vi "Temperature and Humidity Data Acqusition and Logging.vi"() -> ()   [LabVIEW 2017]
uses:
  <vilib>/Instr/_visa.llb/VISA Configure Serial Port (Instr).vi
  <vilib>/Utility/file.llb/Write Delimited Spreadsheet (string).vi
  <vilib>/regexp/Match Regular Expression.xnode
panel:
  out "read buffer":string
  out "Temperature (°F) 2":i32(slide) scale=0.0..300.0
  out "Temperature (°C) 2":i32(slide) scale=0.0..100.0
  in  "Log File Path":path
  in  "Data Table":string[][](table)
  in  "VISA resource name":refnum<visa-resource-name>
  out "Heat Index (°F)":string
  out "Heat Index (°C)":i32(graph)
  out "Temperature (°F)":i32(graph)
  out "Temperature (°C)":i32(graph)
  out "Humidity (%)":i32(graph)
  out "Heat Index (°C)":string
  out "Temperature (°F)":string
  out "Temperature (°C)":string
  out "Humidity (%)":string
  in  "Terminate":bool
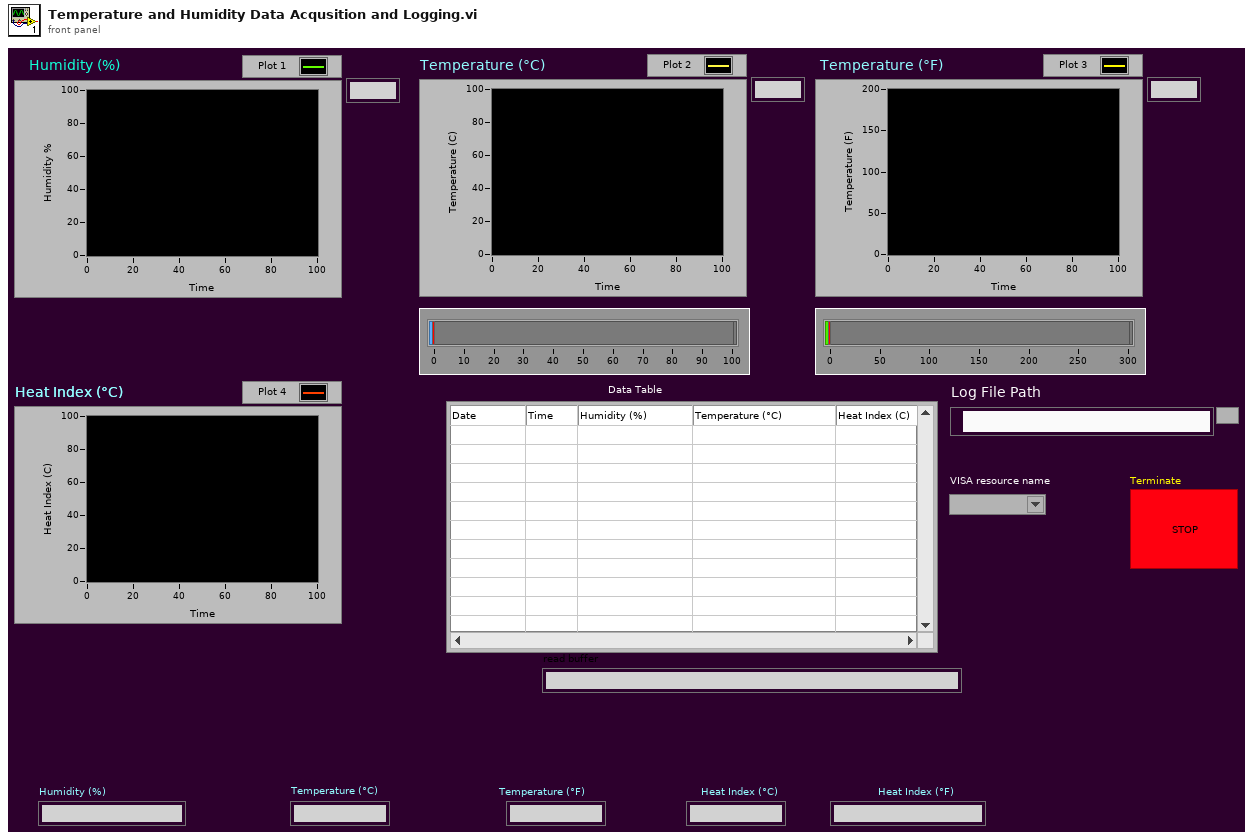
[diagram p1: front panel]
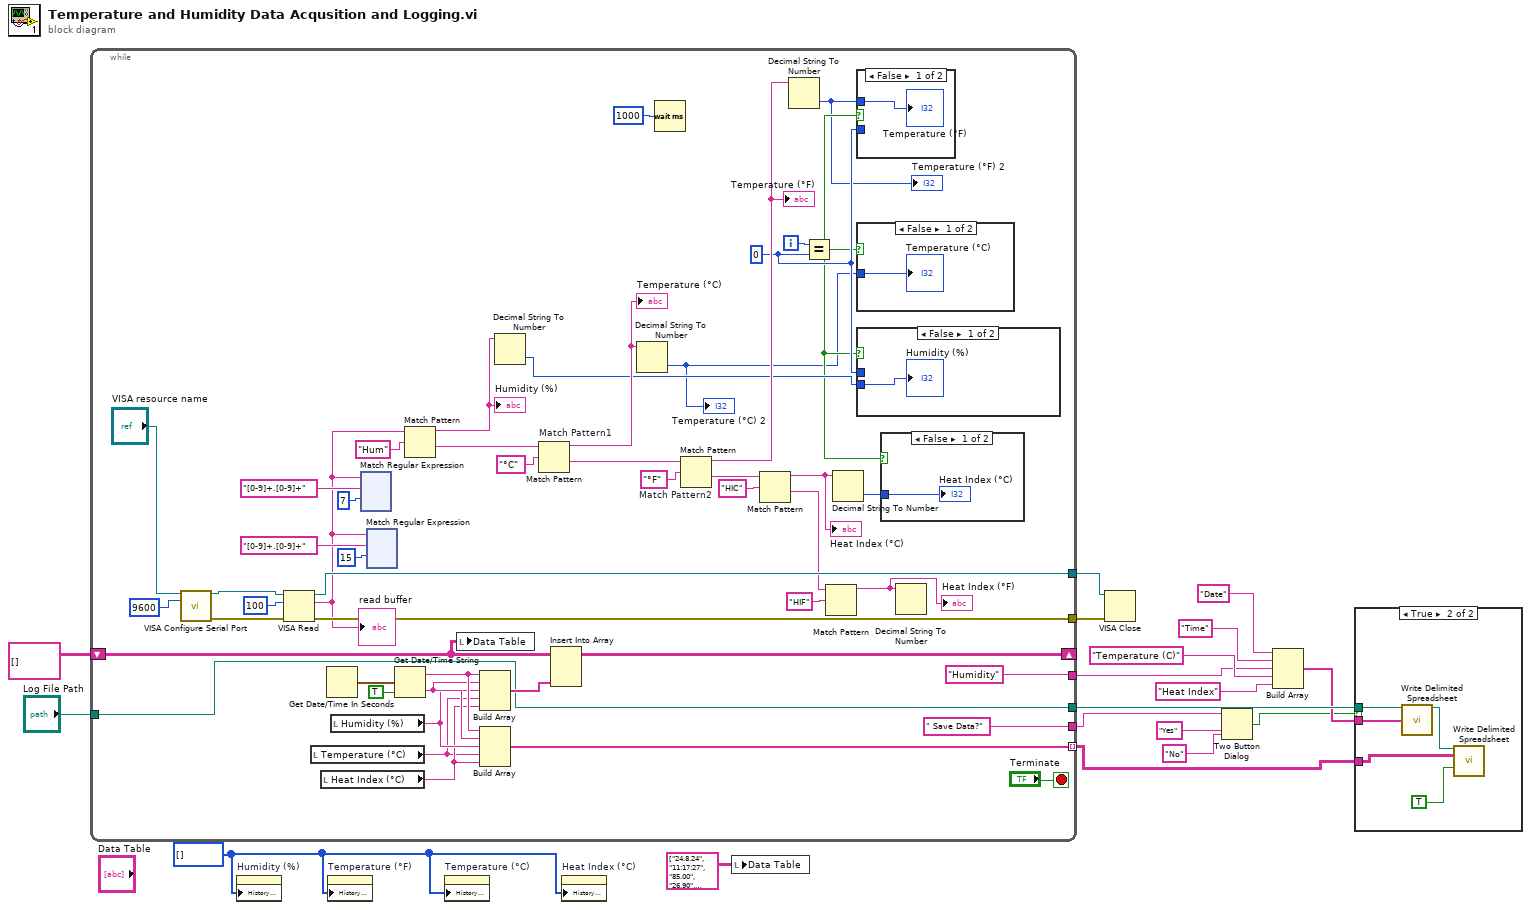
[diagram p0: block diagram]
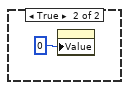
[diagram p3: hidden frame]
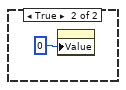
[diagram p4: hidden frame]
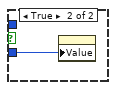
[diagram p5: hidden frame]
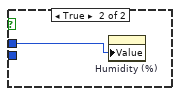
[diagram p6: hidden frame]
diagram:
  w14 = i32[] [] ("History Data")
  n1 = while {
    tunnel: [w50] -> w18
    tunnel: [w49] -> w17
    shift-right: [w29] -> _
    shift-left: string[][] [] -> [w30]
    tunnel: "Log File Path" -> [w22]
    tunnel: [w22] -> w10
    tunnel: ["Humidity" ("regular expression")] -> w8
    tunnel: [" Save Data?" ("regular expression")] -> w4
    tunnel: [w19] -> w2 mode=indexing
    i -> [w28]
    stop <- "Terminate" stop-if-true
    w27 = 0 ("y")
    n2 = call-poly "VISA Configure Serial Port"("VISA resource name"="VISA resource name", "baud rate (9600)"=u32 9600) -> ("VISA resource name out"=w55:refnum<visa-resource-name>, "error out"=w53:errorcluster)  [unwired: 12 in]
    n3 = VISA Read(VISA resource name=w55, byte count=u32 100, error in (no error)=w53) -> (VISA resource name out=w49:refnum<visa-resource-name>, read buffer=w39:string, error out=w50:errorcluster)  [unwired: 1 out]
    "read buffer" <- w39
    n4 = local read "Temperature (°C)"() -> (w25:string)
    n5 = local read "Heat Index (°C)"() -> (w31:string)
    n6 = Get Date/Time In Seconds() -> (seconds since 1Jan1904=w33:timestamp)
    n7 = local read "Humidity (%)"() -> (w32:string)
    n8 = xnode "Match Regular Expression"("input string"=w39, "regular expression"="[0-9]+.[0-9]+", "offset (0)"=7) -> ()  [unwired: 3 in, 5 out]
    n9 = xnode "Match Regular Expression"("input string"=w39, "regular expression"="[0-9]+.[0-9]+", "offset (0)"=15) -> ()  [unwired: 3 in, 5 out]
    n10 = Get Date/Time String(seconds (now)=w33, want seconds? (F)=TRUE) -> (date string=w35:string, time string=w34:string)  [unwired: 1 in]
    n11 = Match Pattern(string=w39, regular expression="Hum") -> (before substring=w63:string, after substring=w42:string)  [unwired: 1 in, 2 out]
    "Humidity (%)" <- w63
    n12 = local write "Data Table"(w30) -> ()
    n13 = Build Array(w35, w34, w32, w25, w31) -> (w37:string[])
    n14 = Build Array(w35, w34, w32, w25, w31) -> (w19:string[])
    n15 = Decimal String To Number(string=w63) -> (number=w38:i32)  [unwired: 2 in, 1 out]
    n16 = Match Pattern "Match Pattern1"(string=w42, regular expression="°C") -> (before substring=w62:string, after substring=w57:string)  [unwired: 1 in, 2 out]
    "Temperature (°C)" <- w62
    n17 = Insert Into Array "Insert Into Array"(array=w30, new element=w37) -> (w29:string[][])  [unwired: 2 in]
    n18 = Decimal String To Number(string=w62) -> (number=w24:i32)  [unwired: 2 in, 1 out]
    "Temperature (°C) 2" <- w24
    n19 = Wait (ms)(milliseconds to wait=u32 1000) -> ()  [unwired: 1 out]
    n20 = Match Pattern "Match Pattern2"(string=w57, regular expression="°F") -> (before substring=w61:string, after substring=w56:string)  [unwired: 1 in, 2 out]
    "Temperature (°F)" <- w61
    n21 = Match Pattern ("Match Pattern1")(string=w56, regular expression="HIC") -> (before substring=w60:string, after substring=w46:string)  [unwired: 1 in, 2 out]
    "Heat Index (°C)" <- w60
    n22 = Decimal String To Number(string=w61) -> (number=w23:i32)  [unwired: 2 in, 1 out]
    "Temperature (°F) 2" <- w23
    n23 = Equal?(x=w28, y=w27) -> (x = y?=w26:bool)
    n24 = Match Pattern ("Match Pattern1")(string=w46, regular expression="HIF") -> (before substring=w45:string)  [unwired: 1 in, 3 out]
    "Heat Index (°F)" <- w45
    n25 = Decimal String To Number(string=w60) -> (number=w58:i32)  [unwired: 2 in, 1 out]
    n26 = case shown="False" w26 {
      tunnel: w23 -> [w72 _]
      tunnel: w27 -> [_ w73]
      frame False {
        "Temperature (°F)" <- w72
      }
      frame True {
        n27 = property on="Temperature (°F)" class="WFChart (strict)"("Value"=w73) -> ()  [unwired: 2 in, 2 out]
      }
    }
    n28 = case shown="False" w26 {
      tunnel: w24 -> [w68 _]
      frame False {
        "Temperature (°C)" <- w68
      }
      frame True {
        n29 = property on="Temperature (°C)" class="WFChart (strict)"("Value"=0 ("y")) -> ()  [unwired: 2 in, 2 out]
      }
    }
    n30 = case shown="False" w26 {
      tunnel: w38 -> [w74 _]
      tunnel: w27 -> [_ w75]
      frame False {
        "Humidity (%)" <- w74
      }
      frame True {
        n31 = property on="Humidity (%)" class="WFChart (strict)"("Value"=w75) -> ()  [unwired: 2 in, 2 out]
      }
    }
    n32 = case shown="False" w26 {
      tunnel: w58 -> [w70 _]
      frame False {
        "Heat Index (°C)" <- w70
      }
      frame True {
        n33 = property on="Heat Index (°C)" class="WFChart (strict)"("Value"=0 ("y")) -> ()  [unwired: 2 in, 2 out]
      }
    }
    n34 = Decimal String To Number(string=w45) -> ()  [unwired: 2 in, 2 out]
  }
  n35 = property on="Humidity (%)" class="WFChart (strict)"("History Data"=w14) -> ()  [unwired: 2 in, 2 out]
  n36 = property on="Temperature (°F)" class="WFChart (strict)"("History Data"=w14) -> ()  [unwired: 2 in, 2 out]
  n37 = property on="Temperature (°C)" class="WFChart (strict)"("History Data"=w14) -> ()  [unwired: 2 in, 2 out]
  n38 = property on="Heat Index (°C)" class="WFChart (strict)"("History Data"=w14) -> ()  [unwired: 2 in, 2 out]
  n39 = local write "Data Table"(string[][] [["24.8.24", "11:17:27", "85.00", "26.90", "29.97"], ["24.8.24", "11:17:28", "830.14HIC86.25HIF\r\n", "", ""], ["24.8.24", "11:17:28", "\r\n", "", ""], ["24.8.24", "11:17:29", "86.00", "26.90", "30.14"], ["24.8.24", "11:17:29", "86.00", "26.90", "30.14"], ["24.8.24", "11:17:30", "86.00", "26.90", "30.14"], ["24.8.24", "11:17:30", "86.00", "26.90", "30.14"], ["24.8.24", "11:17:32", "86.00", "26.90", "30.14"], ["24.8.24", "11:17:34", "86.00", "26.80", "29.89"], ["24.8.24", "11:17:36", "86.00", "26.80", "29.89"], ["24.8.24", "11:17:38", "86.00", "26.80", "29.89"], ["24.8.24", "11:17:40", "86.00", "26.80", "29.89"], ["24.8.24", "11:17:42", "86.00", "26.80", "29.89"], ["24.8.24", "11:17:44", "86.00", "26.80", "29.89"], ["24.8.24", "11:17:46", "86.00", "26.80", "29.89"], ["24.8.24", "11:17:48", "86.00", "26.80", "29.89"], ["24.8.24", "11:17:50", "86.00", "26.80", "29.89"], ["24.8.24", "11:17:52", "86.00", "26.80", "29.89"], ["24.8.24", "11:17:54", "86.00", "26.90", "30.14"], ["24.8.24", "11:17:56", "86.00", "26.80", "29.89"], ["24.8.24", "11:17:58", "85.00", "26.80", "29.73"]] ("Data Table")) -> ()
  n40 = VISA Close(VISA resource name=w17, error in (no error)=w18) -> ()  [unwired: 1 out]
  n41 = Two Button Dialog(message=w4, 1:"No" ("F button name (\"Cancel\")"), 2:"Yes" ("T button name (\"OK\")")) -> (T button?=w3:bool)
  n42 = Build Array("Date" ("regular expression"), "Time" ("regular expression"), w8, "Temperature (C)" ("regular expression"), "Heat Index" ("element")) -> (w9:string[])
  n43 = case shown="True" w3 {
    tunnel: w10 -> [_ w308]
    tunnel: w9 -> [_ w307]
    tunnel: w2 -> [_ w305]
    frame False {
    }
    frame True {
      n44 = call-poly <vilib>:"Write Delimited Spreadsheet.vi"("file path (dialog if empty)"=w308, "1D data"=w307) -> ("new file path (Not A Path if cancelled)"=w304:path)  [unwired: 12 in, 1 out]
      n45 = call-poly <vilib>:"Write Delimited Spreadsheet.vi"("file path (dialog if empty)"=w304, "2D data"=w305, "append to file? (new file:F)"=TRUE) -> ()  [unwired: 11 in, 2 out]
    }
  }
